vi "纳清_第一点校准数据写入.vi"(7 "探头":T1(ring), 8 "error in (no error)":errorcluster caption="错误输入（无错误）", 10 "数值":sgl, 11 "MB session in":refnum<class "MB_Master.lvclass">) -> (0 "error out":errorcluster caption="错误输出", 3 "MB session out":refnum<class "MB_Master.lvclass">)   [LabVIEW 2016, in "斯坦道多参数.lvlib"]
uses:
  <vilib>/Plasmionique/MB Master/MB_Master/MB_Master.lvclass
  <vilib>/Plasmionique/MB Master/MB Master.lvlib
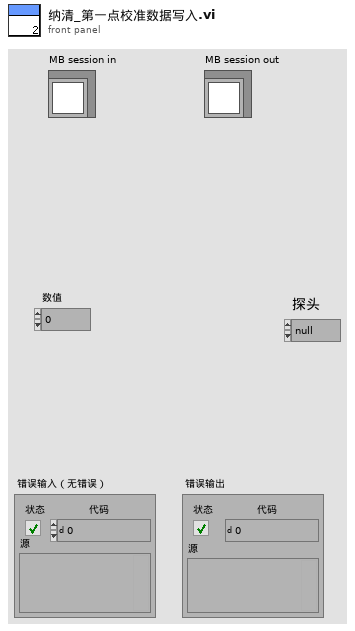
[diagram p1: front panel]
types:
  T1 = enum16{"null", "pH", "DO", "浊度", "电导率", "叶绿素a", "藻密度"}
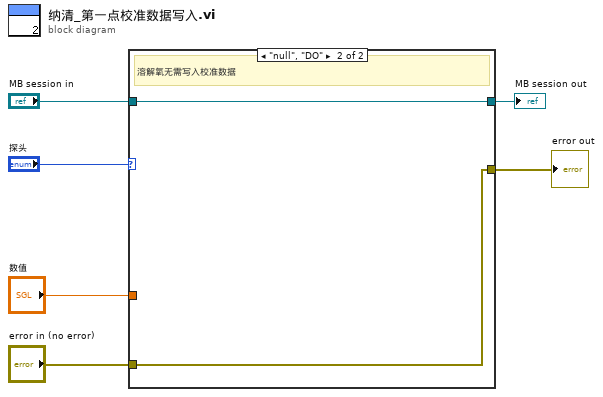
[diagram p0: block diagram]
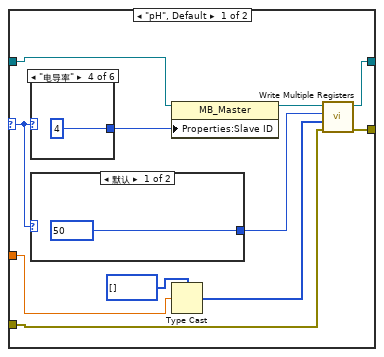
[diagram p2: hidden frame]
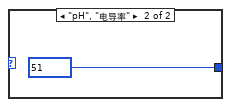
[diagram p3: hidden frame]
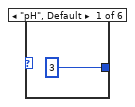
[diagram p4: hidden frame]
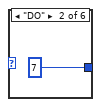
[diagram p5: hidden frame]
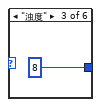
[diagram p6: hidden frame]
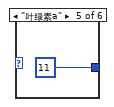
[diagram p7: hidden frame]
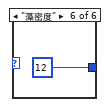
[diagram p8: hidden frame]
diagram:
  n1 = case shown="\"null\", \"DO\"" "探头" {
    selector: "探头" -> [w7 _]
    tunnel: "error in (no error)" -> [w17 w26]
    tunnel: [w16 w26] -> w5
    tunnel: "数值" -> [w14 _]
    tunnel: "MB session in" -> [w11 w27]
    tunnel: [w10 w27] -> w2
    frame "pH", Default {
      n2 = case shown="\"电导率\"" w7 {
        tunnel: [3 7 8 4 11 12] -> w9
        frame "pH", Default {
        }
        frame "DO" {
        }
        frame "浊度" {
        }
        frame "电导率" {
        }
        frame "叶绿素a" {
        }
        frame "藻密度" {
        }
      }
      n3 = case shown="默认" w7 {
        tunnel: [u16 50 ("starting address") u16 51 ("starting address")] -> w8
        frame Default {
        }
        frame "pH", "电导率" {
        }
      }
      n4 = property class="MB_Master"(reference=w11, "Properties:Slave ID"=w9) -> (reference out=w15:refnum<class "MB_Master.lvclass">)  [unwired: 1 in, 1 out]
      n5 = Type Cast(type=u16[] [], x=w14) -> (*(type *) &x=w12:u16[])
      n6 = call <vilib>:"Write Multiple Registers.vi"("error in (no error)"=w17, "values"=w12, "starting address"=w8, "MB session in"=w15) -> ("error out"=w16:errorcluster, "MB session out"=w10:refnum<class "MB_Master.lvclass">)  [unwired: 6 in]
    }
    frame "null", "DO" {
      # "溶解氧无需写入校准数据"
    }
  }
  "error out" <- w5
  "MB session out" <- w2
